vi "Get t0 on Variant.vi"(8 "error in (no error)":errorcluster, 11 "Variant in":variant) -> (0 "error out":errorcluster, 2 "t0":timestamp, 3 "Variant out":variant)   [LabVIEW 2020, in "Internal Comm Classes.lvlib" / "WPL Comm.lvclass"]
uses:
  WPL Comm.lvclass
  <vilib>/Utility/error.llb/Error Cluster From Error Code.vi
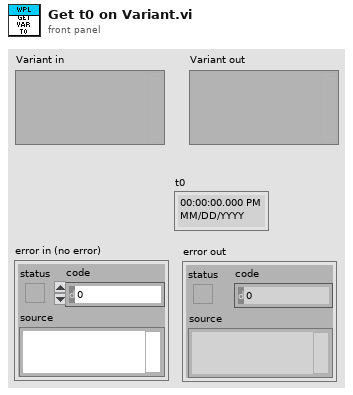
[diagram p1: front panel]
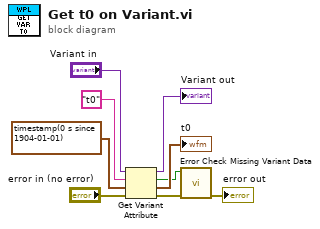
[diagram p0: block diagram]
diagram:
  n1 = Get Variant Attribute(Variant="Variant in", name="t0", default value (empty Variant)=timestamp(0 s since 1904-01-01) ("t0"), error in="error in (no error)") -> (duplicate Variant=→"Variant out":variant, found=w3:bool, value=→"t0":timestamp, error out=w2:errorcluster)
  n2 = call "Error Check Missing Variant Data.vi"("error in (no error)"=w2, "Found?"=w3) -> ("error out"=→"error out":errorcluster)  [unwired: 9 in]
